vi "搜索ID.vi"(0 "Array":string[][](array[string]), 1 "ID选择":enum16{"旧ID", "新ID"}(ring), 5 "LOtID":string, 7 "WaferID":string, 9 "DieID":string, 11 "error in":errorcluster) -> (6 "ID?":bool, 8 "Numeric":i32, 15 "error out":errorcluster)   [LabVIEW 2016]
panel:
  out "array w/ subset deleted":string[][](array[string])
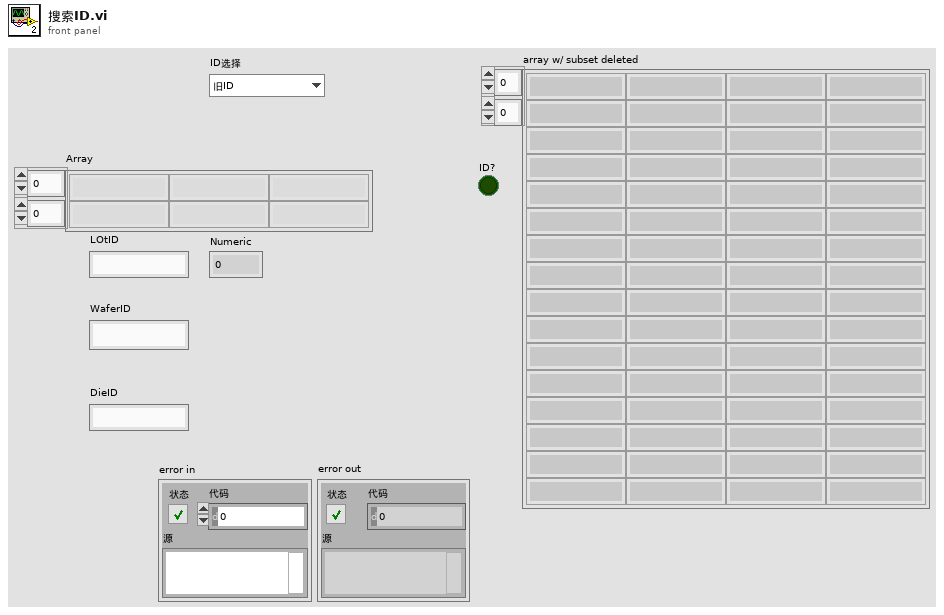
[diagram p1: front panel]
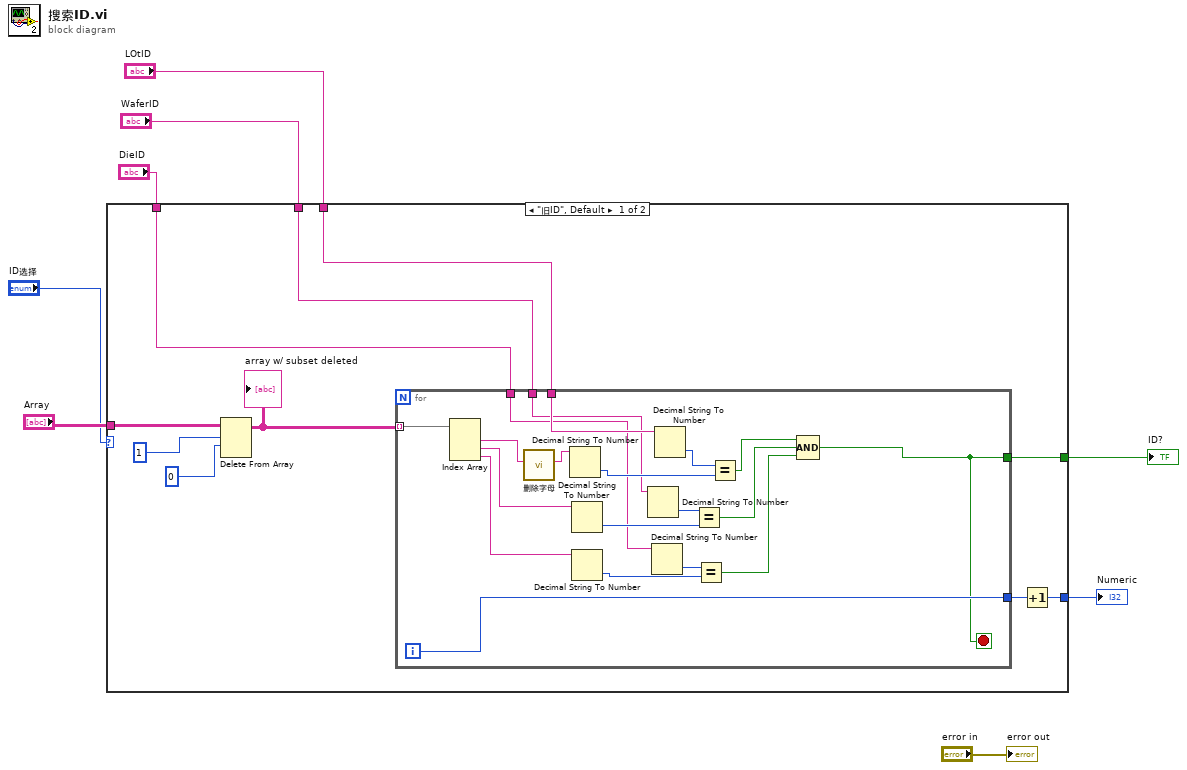
[diagram p0: block diagram]
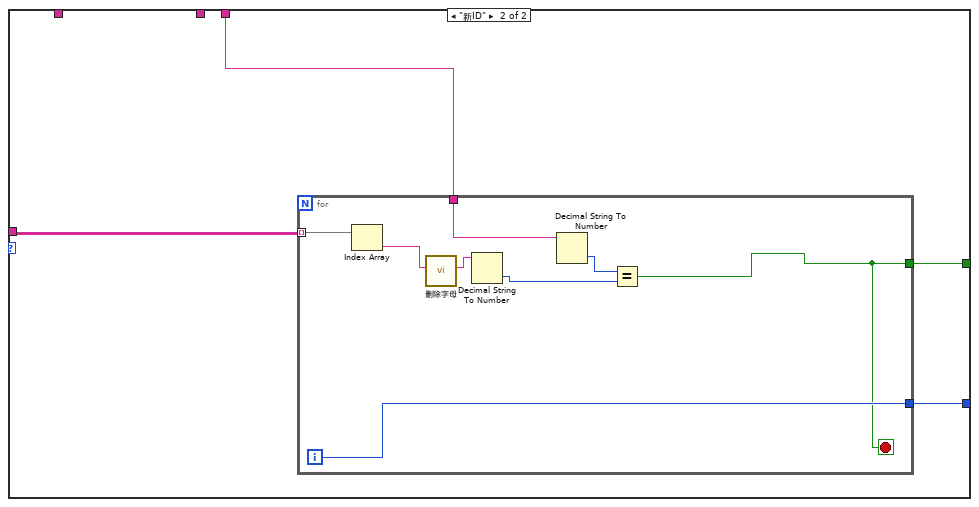
[diagram p2: hidden frame]
diagram:
  n1 = case shown="\"旧ID\", Default" "ID选择" {
    tunnel: [w18 w41] -> w8
    tunnel: "Array" -> [w17 w38]
    tunnel: [w9 w40] -> w1
    tunnel: "LOtID" -> [w13 w39]
    tunnel: "WaferID" -> [w12 _]
    tunnel: "DieID" -> [w11 _]
    frame "旧ID", Default {
      n2 = Delete From Array(array=w17, length=1, index (row)=0) -> (array with subset deleted=w14:string[][])  [unwired: 1 in, 1 out]
      "array w/ subset deleted" <- w14
      n3 = for {
        tunnel: w14 -> [w37] mode=indexing
        tunnel: w13 -> [w36]
        tunnel: w12 -> [w32]
        tunnel: w11 -> [w28]
        tunnel: [w19] -> w18
        tunnel: [w22] -> w10
        i -> [w22]
        stop <- w19 stop-if-true
        n4 = Index Array(array=w37) -> (element #1=w21:string, element #2=w33:string, element #3=w29:string)  [unwired: 3 in]
        n5 = call "删除字母.vi"("输入字符串"=w21) -> ("输出字符串"=w20:string)  [unwired: 10 in]
        n6 = Decimal String To Number(string=w20) -> (number=w34:i32)  [unwired: 2 in, 1 out]
        n7 = Decimal String To Number(string=w33) -> (number=w30:i32)  [unwired: 2 in, 1 out]
        n8 = Decimal String To Number(string=w29) -> (number=w26:i32)  [unwired: 2 in, 1 out]
        n9 = Decimal String To Number(string=w32) -> (number=w31:i32)  [unwired: 2 in, 1 out]
        n10 = Decimal String To Number(string=w28) -> (number=w27:i32)  [unwired: 2 in, 1 out]
        n11 = Decimal String To Number(string=w36) -> (number=w35:i32)  [unwired: 2 in, 1 out]
        n12 = Equal?(x=w31, y=w30) -> (x = y?=w24:bool)
        n13 = Equal?(x=w27, y=w26) -> (x = y?=w23:bool)
        n14 = Equal?(x=w35, y=w34) -> (x = y?=w25:bool)
        n15 = Compound Arithmetic op=AND(w25, w24, w23) -> (w19:bool)
      }
      n16 = Increment(x=w10) -> (x+1=w9:i32)
    }
    frame "新ID" {
      n17 = for {
        tunnel: w38 -> [w49] mode=indexing
        tunnel: w39 -> [w48]
        tunnel: [w42] -> w41
        tunnel: [w45] -> w40
        i -> [w45]
        stop <- w42 stop-if-true
        n18 = Index Array(array=w49) -> (element=w44:string)  [unwired: 1 in]
        n19 = call "删除字母.vi"("输入字符串"=w44) -> ("输出字符串"=w43:string)  [unwired: 10 in]
        n20 = Decimal String To Number(string=w43) -> (number=w46:i32)  [unwired: 2 in, 1 out]
        n21 = Decimal String To Number(string=w48) -> (number=w47:i32)  [unwired: 2 in, 1 out]
        n22 = Equal?(x=w47, y=w46) -> (x = y?=w42:bool)
      }
    }
  }
  "ID?" <- w8
  "Numeric" <- w1
  "error out" <- "error in"
